vi "LeCroy.Configure Time.vi"(8 "Error In":errorcluster, 9 "Sample Points":i32(ring)=500 items=["50"=50, "100"=100, "250"=250, "500"=500, "1000"=1000, "2500"=2500, "5K"=5000, "10K"=10000, "25K"=25000, "50K"=50000, "100K"=100000, "250K"=250000, "500K"=500000, "1M"=1000000, "2M"=2000000, "2.5M"=2500000, "5M"=5000000, "10M"=10000000, "25M"=25000000, "50M"=50000000, "100M"=100000000], 10 "Timebase":dbl=0.0005, 11 "LeCroy.Session in":T1) -> (0 "Error Out":errorcluster, 3 "LeCroy.Session out":T1)   [LabVIEW 2018]
uses:
  typedefs/LeCroy.Session.ctl
  <instrlib>/LeCroy Wave Series/LeCroy Wave Series.lvlib
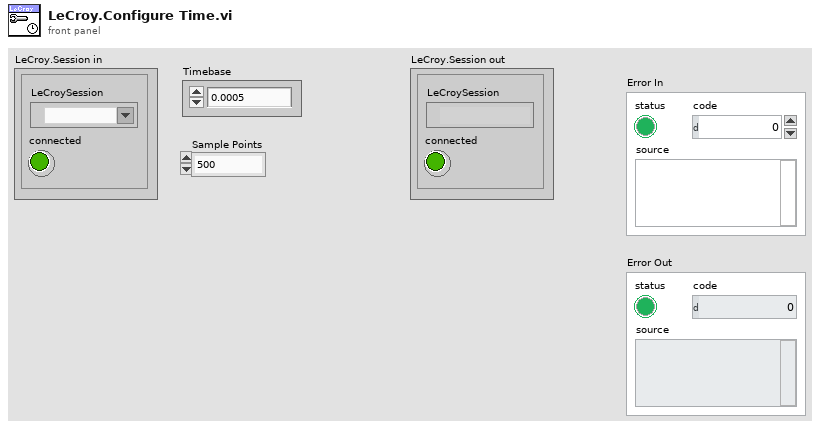
[diagram p1: front panel]
types:
  T1 = typedef "LeCroy.Session.ctl" = cluster{"LeCroySession":refnum<visa-resource-name>, "connected":bool}
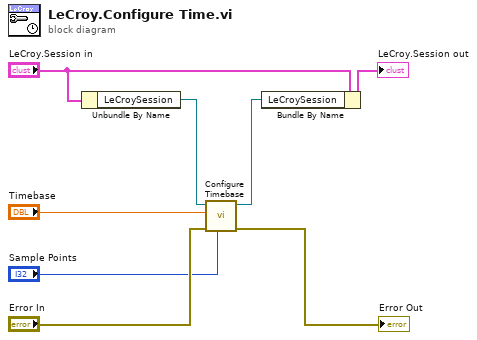
[diagram p0: block diagram]
diagram:
  n1 = Unbundle By Name("LeCroy.Session in") -> ("LeCroySession"=w6:refnum<visa-resource-name>)
  n2 = call <instrlib>:"Configure Timebase.vi"("Maximum Sample Points (500)"="Sample Points", "error in (no error)"="Error In", "Timebase (0.0005 s)"="Timebase", "VISA resource name"=w6) -> ("error out"=→"Error Out":errorcluster, "VISA resource name out"=w5:refnum<visa-resource-name>)  [unwired: 6 in]
  n3 = Bundle By Name(cluster="LeCroy.Session in", "LeCroySession"=w5) -> (→"LeCroy.Session out":T1)
